vi "测试.vi"(5 "I-V扫描":T2, 6 "功能选择":u16(ring) items=["I-V扫描", "脉冲测试", "维持时间"], 7 "脉冲测试":T1, 8 "错误输入":errorcluster, 10 "维持时间":T3, 11 "VISA资源名称":refnum<visa-resource-name>) -> (0 "错误输出":errorcluster, 3 "VISA资源名称输出":refnum<visa-resource-name>)   [LabVIEW 2019]
uses:
  lib/Global variable.vi
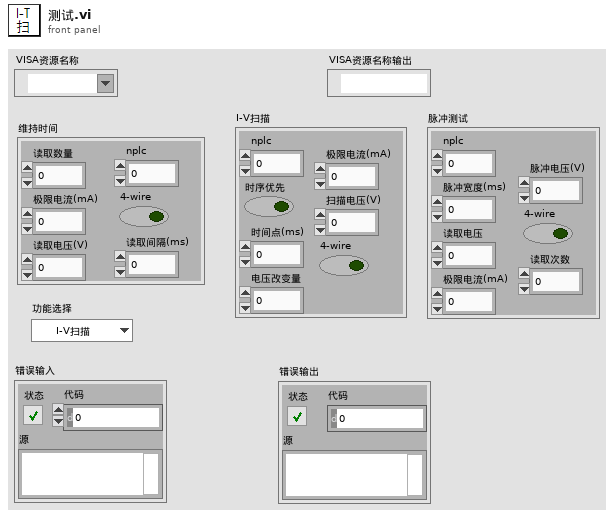
[diagram p1: front panel]
types:
  T1 = cluster{"nplc":dbl, "脉冲宽度(ms)":dbl, "读取电压":dbl, "极限电流(mA)":dbl, "脉冲电压(V)":dbl, "4-wire":bool, "读取次数":dbl}
  T2 = cluster{"nplc":dbl, "时序优先":bool, "时间点(ms)":dbl, "电压改变量":dbl, "极限电流(mA)":dbl, "扫描电压(V)":dbl, "4-wire":bool}
  T3 = cluster{"nplc":dbl, "4-wire":bool, "读取间隔(ms)":dbl, "读取数量":dbl, "极限电流(mA)":dbl, "读取电压(V)":dbl}
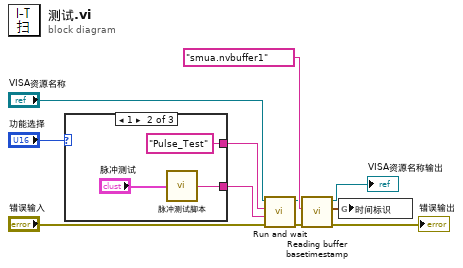
[diagram p0: block diagram]
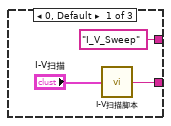
[diagram p2: hidden frame]
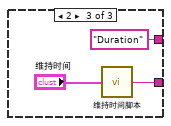
[diagram p3: hidden frame]
diagram:
  n1 = case shown="1" "功能选择" {
    tunnel: [w14 w16 w20] -> w3
    tunnel: ["I_V_Sweep" ("Script Name") "Pulse_Test" ("Script Name") "Duration" ("Script Name")] -> w1
    frame 0, Default {
      n2 = call "I-V扫描脚本.vi"("参数"="I-V扫描") -> ("Script"=w14:string)
    }
    frame 1 {
      n3 = call "脉冲测试脚本.vi"("参数"="脉冲测试") -> ("Script"=w16:string)
    }
    frame 2 {
      n4 = call "维持时间脚本.vi"("参数"="维持时间") -> ("Script"=w20:string)
    }
  }
  n5 = call "Run and wait.vi"("错误输入"="错误输入", "Script"=w3, "Script Name"=w1, "VISA资源名称"="VISA资源名称") -> ("错误输出"=w8:errorcluster, "VISA资源名称输出"=w9:refnum<visa-resource-name>)  [unwired: 6 in]
  n6 = call "Reading buffer basetimestamp.vi"("错误输入"=w8, "缓冲区名称"="smua.nvbuffer1", "VISA资源名称"=w9) -> ("错误输出"=→"错误输出":errorcluster, "时间标识"=w11:timestamp, "VISA资源名称输出"=→"VISA资源名称输出":refnum<visa-resource-name>)  [unwired: 6 in]
  n7 = global write "Global variable.vi" "时间标识"(w11) -> ()
